vi "Variant Tools Test.vi"() -> ()   [LabVIEW 2013, in "JSONtext.lvlib"]
uses:
  JSONtext.lvlib
panel:
  out "length":i32
  out "Variant out":variant
  out "To Variant":dbl[](array[numeric]) format="%#_3p"
  in  "Cluster":T1={"A 6"=34, "T 1"="Line 1", "A"=34, "<JSON>T 3"="{\"T\":123}", "T 4"="sdfsdfdsfsdf", "A 2"=1.23456, "T 5"="Test \"quote\",\nand newline.", "T 6"="sdfsdf", "A 3"=34, "Cluster 2"={"T 1"="SubCluster", "T 2"="Test \"quote\",\nand newline.", "A"=34, "T 3"="Test \"quote\",\nand newline.", "T 4"="Test \"quote\",\nand newline.", "A 2"=34, "T 5"="Test \"quote\",\nand newline.", "T 6"="Test \"quote\",\nand newline.", "A 3"=34}, "Array"=array[100001 elements]}
  out "x = y?":bool
  out "<JSON>":string
  out "error out":errorcluster
  out "data":T2={"<JSON>Cluster 2"="Test \"dfsdfsdfd\",\nand newline.", "T 1"="Line 1", "A 2"=1.23456}
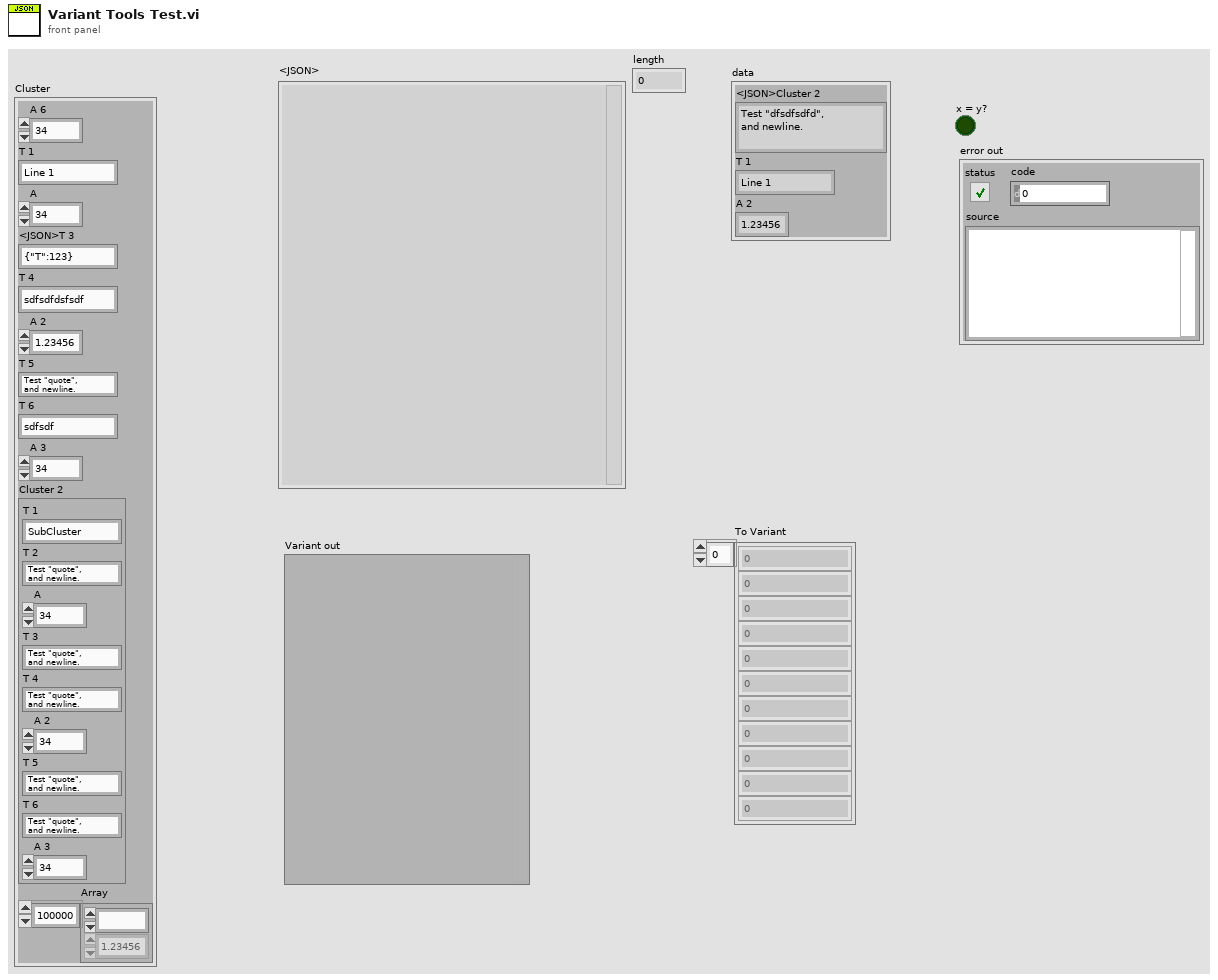
[diagram p1: front panel]
types:
  T1 = cluster{"A 6":i32, "T 1":string, "A":i32, "<JSON>T 3":string, "T 4":string, "A 2":dbl, "T 5":string, "T 6":string, "A 3":i32, "Cluster 2":cluster{"T 1":string, "T 2":string, "A":i32, "T 3":string, "T 4":string, "A 2":i32, "T 5":string, "T 6":string, "A 3":i32}, "Array":dbl[]}
  T2 = cluster{"<JSON>Cluster 2":string, "T 1":string, "A 2":dbl}
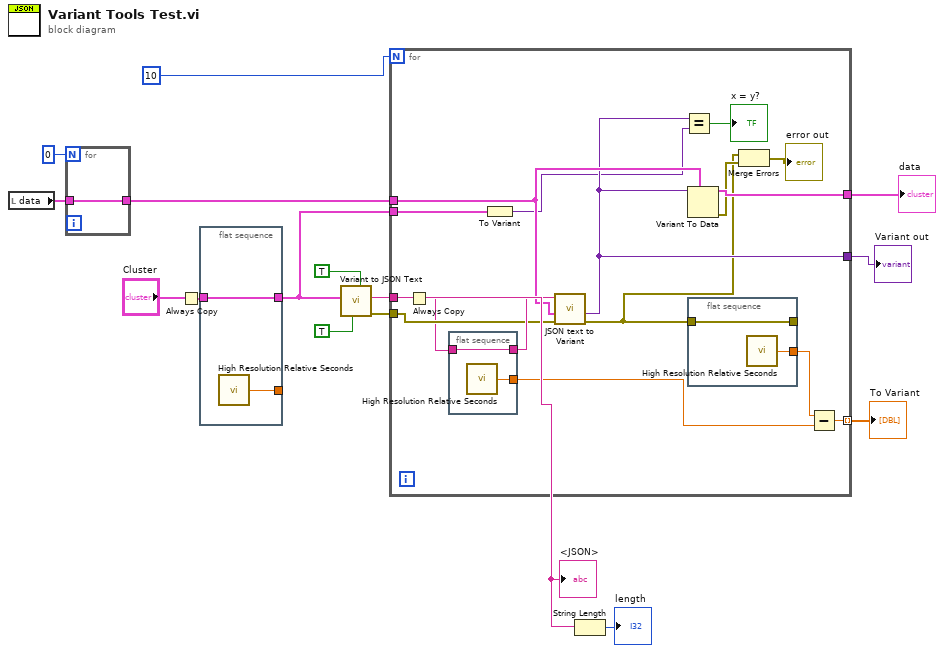
[diagram p0: block diagram]
diagram:
  n1 = local read "data"() -> (w11:T2)
  n2 = for {
    N: 0 -> [_]
    tunnel: [w16] -> w12
    tunnel: w11 -> [w16]
  }
  n3 = Always Copy(1:"Cluster") -> (0:w2:T1)
  n4 = flat-sequence {
    tunnel: w2 -> [w17]
    tunnel: [w18] -> _
    tunnel: [w17] -> w4
    frame #0 {
      n5 = call <vilib>:"High Resolution Relative Seconds.vi"() -> ("relative seconds"=w18:dbl)
    }
  }
  n6 = call "Variant to JSON Text.vi"("enable LabVIEW extensions? (T)"=TRUE, "Pretty Print?"=TRUE, "Variant"=w4) -> ("error out"=w3:errorcluster, "<JSON>"=w9:string)  [unwired: 7 in]
  "<JSON>" <- w9
  n7 = for {
    N: 10 -> [_]
    tunnel: [w34] -> w14 mode=indexing
    tunnel: w12 -> [w33]
    tunnel: w9 -> [w22]
    tunnel: [w32] -> w8
    tunnel: [w31] -> w7
    tunnel: w4 -> [w26]
    tunnel: w3 -> [w20]
    n8 = Always Copy(1:w22) -> (0:w19:string)
    n9 = flat-sequence {
      tunnel: [w36] -> w21
      tunnel: w19 -> [w36]
      tunnel: [w35] -> w25
      frame #0 {
        n10 = call <vilib>:"High Resolution Relative Seconds.vi"() -> ("relative seconds"=w35:dbl)
      }
    }
    n11 = To Variant(anything=w26) -> (Variant=w29:variant)
    n12 = call "JSON text to Variant.vi"("error in (no error)"=w20, "Variant (Data Type)"=w33, "JSON"=w21) -> ("error out"=w23:errorcluster, "Variant out"=w31:variant)  [unwired: 7 in]
    n13 = Equal?(x=w31, y=w29) -> (x = y?=→"x = y?":bool)
    n14 = Variant To Data(type=w33, Variant=w31) -> (data=w32:T2, error out=w30:errorcluster)  [unwired: 1 in]
    n15 = flat-sequence {
      tunnel: [w38] -> _
      tunnel: w23 -> [w38]
      tunnel: [w37] -> w27
      frame #0 {
        n16 = call <vilib>:"High Resolution Relative Seconds.vi"() -> ("relative seconds"=w37:dbl)
      }
    }
    n17 = Merge Errors(w23, w30) -> (→"error out":errorcluster)
    n18 = Subtract(x=w27, y=w25) -> (x-y=w34:dbl)
  }
  "To Variant" <- w14
  "data" <- w8
  "Variant out" <- w7
  n19 = String Length(string=w9) -> (length=→"length":i32)
